vi "Send Data to Controller.vi"(10 "notifier in":refnum<notifier>, 11 "Device in":refnum<class "Device.lvclass">) -> ()   [LabVIEW 2014, in "DAQ Device.lvlib" / "Device.lvclass"]
uses:
  Device.lvclass
  <vilib>/ActorFramework/Actor/Actor.lvclass/Actor.ctl
  Device.lvclass/Device.ctl
  Devices/Configurable Device/Configurable Device.lvclass/Configurable Device.ctl
  Generic Data Update Data MSG/Generic Update Data Message.lvclass/Generic Update Data Message.ctl
  <vilib>/ActorFramework/Message Enqueuer/Message Enqueuer.lvclass/Message Enqueuer.ctl
  Generic Data Update Data MSG/Write Data.vi
  Devices/Configurable Device/Read ID.vi
  Generic Data Update Data MSG/Write ID.vi
  <vilib>/ActorFramework/Message Priority Queue/Priority Enqueue.vi
  Devices/Configurable Device/Configurable Device.lvclass
  <vilib>/ActorFramework/Message Enqueuer/Message Enqueuer.lvclass
  <vilib>/ActorFramework/Actor/Actor.lvclass
  Generic Data Update Data MSG/Generic Update Data Message.lvclass
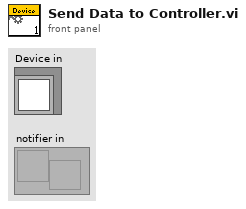
[diagram p1: front panel]
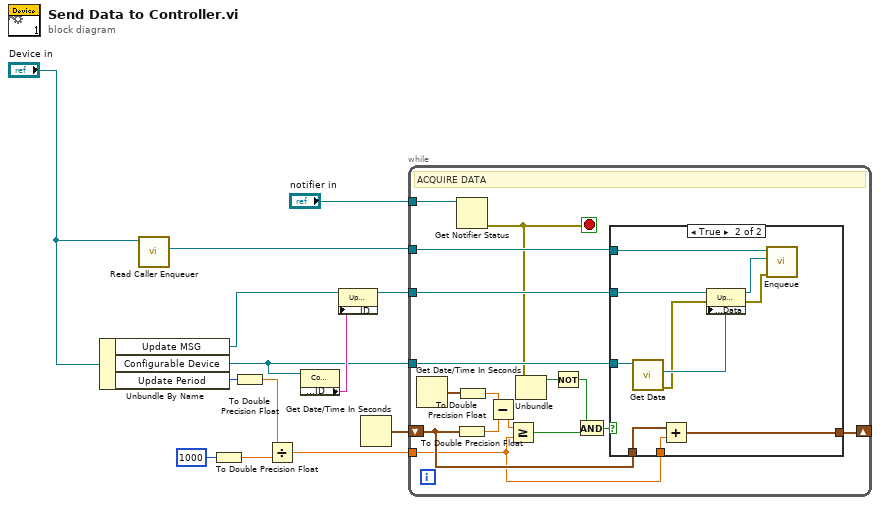
[diagram p0: block diagram]
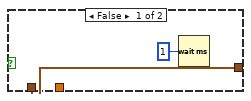
[diagram p2: hidden frame]
diagram:
  n1 = Unbundle By Name("Device in") -> ("Update MSG"=w10:refnum<class "Generic Update Data Message.lvclass">, "Configurable Device"=w5:refnum<class "Configurable Device.lvclass">, "Update Period"=w6:i32)
  n2 = call <vilib>:"Read Caller Enqueuer.vi"("Actor"="Device in") -> ("Caller Enqueuer"=w4:refnum<class "Message Enqueuer.lvclass">)  [unwired: 10 in]
  n3 = To Double Precision Float(number=1000 ("y")) -> (double precision float=w8:dbl)
  n4 = To Double Precision Float(number=w6) -> (double precision float=w7:dbl)
  n5 = Divide(x=w7, y=w8) -> (x/y=w2:dbl)
  n6 = property class="Configurable Device"(reference=w5) -> ("Accessors:ID"=w12:string)  [unwired: 1 in, 2 out]
  n7 = property class="Update Data MSG"(reference=w10, "Accessors:ID"=w12) -> (reference out=w11:refnum<class "Generic Update Data Message.lvclass">)  [unwired: 1 in, 1 out]
  n8 = Get Date/Time In Seconds() -> (seconds since 1Jan1904=w1:timestamp)
  n9 = while {
    tunnel: w4 -> [w29]
    tunnel: w5 -> [w28]
    shift-right: [w21] -> _
    shift-left: w1 -> [w23]
    tunnel: w2 -> [w22]
    tunnel: "notifier in" -> [w20]
    tunnel: w11 -> [w19]
    stop <- w18 stop-if-true
    # "ACQUIRE DATA"
    n10 = Get Date/Time In Seconds() -> (seconds since 1Jan1904=w27:timestamp)
    n11 = Get Notifier Status(notifier=w20) -> (error out=w18:errorcluster)  [unwired: 1 in, 4 out]
    n12 = To Double Precision Float(number=w23) -> (double precision float=w25:dbl)
    n13 = To Double Precision Float(number=w27) -> (double precision float=w26:dbl)
    n14 = Subtract(x=w26, y=w25) -> (x-y=w24:dbl)
    n15 = Greater Or Equal?(x=w24, y=w22) -> (x >= y?=w15:bool)
    n16 = Unbundle(w18) -> ("status"=w17:bool)  [unwired: 2 out]
    n17 = Not(x=w17) -> (.not. x?=w16:bool)
    n18 = And(x=w16, y=w15) -> (x .and. y?=w14:bool)
    n19 = case shown="True" w14 {
      tunnel: w29 -> [_ w41]
      tunnel: w28 -> [_ w40]
      tunnel: w23 -> [w31 w39]
      tunnel: w22 -> [_ w38]
      tunnel: [w31 w37] -> w21
      tunnel: w19 -> [_ w36]
      frame False {
        n20 = Wait (ms)(milliseconds to wait=u32 1) -> ()  [unwired: 1 out]
      }
      frame True {
        n21 = call-dynamic "Get Data.vi"("Configurable Device in"=w40) -> ("error out"=w33:errorcluster, "DataOut"=w35:refnum<class "Data.lvclass">)  [unwired: 8 in, 1 out]
        n22 = Add(x=w39, y=w38) -> (x+y=w37:timestamp)
        n23 = property class="Update Data MSG"(reference=w36, error in=w33, "Accessors:Data"=w35) -> (reference out=w34:refnum<class "Generic Update Data Message.lvclass">, error out=w32:errorcluster)
        n24 = call <vilib>:"Enqueue.vi"("error in (no error)"=w32, "Message"=w34, "Message Enqueuer in"=w41) -> ()  [unwired: 7 in, 2 out]
      }
    }
  }
